vi "Add item.vi"(9 "Value":refnum<class "IMessagePackObject.lvclass">, 10 "Key":refnum<class "IMessagePackObject.lvclass">, 11 "MsgPackMap in":refnum<class "MsgPackMap.lvclass">) -> (3 "MsgPackMap out":refnum<class "MsgPackMap.lvclass">)   [LabVIEW 2020, in "MessagePack.lvlib" / "MsgPackMap.lvclass"]
uses:
  MsgPackMap.lvclass
  IMessagePackObject/IMessagePackObject.lvclass
  MsgPackMap.lvclass/MsgPackMap.ctl
  <vilib>/Utility/miscctls.llb/LVMapReplaceAction.ctl
panel:
  out "value unchanged?":bool
  out "key already included?":bool
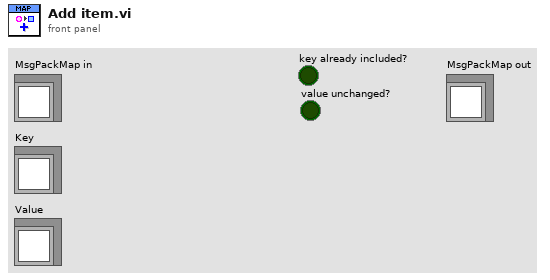
[diagram p1: front panel]
types:
  T1 = typedef "LVMapReplaceAction.ctl" = enum32{"Modify Entry only if found", "Add or Modify Entry", "Delete Entry"}
  T2 = map{refnum<class "IMessagePackObject.lvclass">, refnum<class "IMessagePackObject.lvclass">}
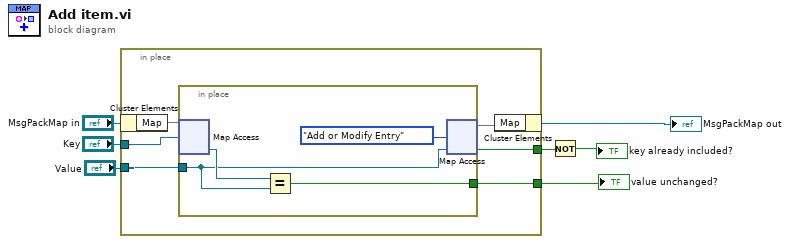
[diagram p0: block diagram]
diagram:
  n1 = in-place {
    in-place-border: "Key" -> [w11]
    in-place-border: "Value" -> [w10]
    in-place-border: [w9] -> w3
    in-place-border: [w8] -> w1
    n2 = in-place-cluster #1("MsgPackMap in") -> ("Map"=w13:T2)
    n3 = in-place {
      in-place-border: w10 -> [w15]
      in-place-border: [w14] -> w8
      n4 = in-place-map #2(w13, w11) -> (w16:refnum<class "IMessagePackObject.lvclass">)  [unwired: 1 in, 1 out]
      n5 = Equal?(x=w16, y=w15) -> (x = y?=w14:bool)
      n6 = in-place-map #2(w15, LVMapReplaceAction."Add or Modify Entry" ("action")) -> (w12:T2, w9:bool)  [unwired: 1 out]
    }
    n7 = in-place-cluster #1("Map"=w12) -> (→"MsgPackMap out":refnum<class "MsgPackMap.lvclass">)
  }
  "value unchanged?" <- w1
  n8 = Not(x=w3) -> (.not. x?=→"key already included?":bool)
